vi "log pelco cmd 2 (SubVI).vi"(10 "Enum(log)":enum16{"Log", "Init"}(ring), 11 "String":string) -> (3 "Cam rcv":string)   [LabVIEW 2018]
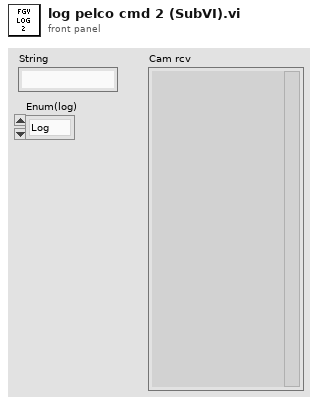
[diagram p1: front panel]
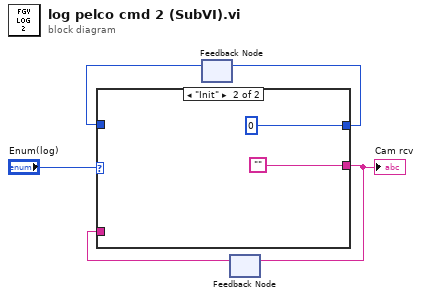
[diagram p0: block diagram]
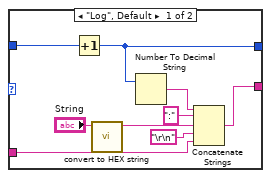
[diagram p2: hidden frame]
diagram:
  n1 = feedback #1() -> (w3:i32)  [unwired: 1 in]
  n2 = feedback #2() -> (w1:string)  [unwired: 1 in]
  n3 = case shown="\"Init\"" "Enum(log)" {
    tunnel: [w7 ""] -> w2
    tunnel: [w9 0] -> w4
    tunnel: w3 -> [w8 _]
    tunnel: w1 -> [w6 _]
    frame "Log", Default {
      n4 = Increment(x=w8) -> (x+1=w9:i32)
      n5 = call "convert to HEX string.vi"("String In(binary)"="String") -> ("String Out (hexa)"=w14:string)  [unwired: 10 in]
      n6 = Number To Decimal String(number=w9) -> (decimal integer string=w13:string)  [unwired: 1 in]
      n7 = Concatenate Strings(w13, ":" ("string"), w14, "\r\n", w6) -> (w7:string)
    }
    frame "Init" {
    }
  }
  "Cam rcv" <- w2
  n8 = feedback-in #1(w4) -> ()
  n9 = feedback-in #2(w2) -> ()
